vi "Get Plugin Paths.vi"(8 "error in":errorcluster, 11 "measurement customizations in":refnum<class "Measurement Plugin.lvclass">) -> (0 "error out":errorcluster, 2 "plugin paths":T1, 3 "measurement customizations out":refnum<class "Measurement Plugin.lvclass">)   [LabVIEW 2021, in "NIDAQmxMeasurement.lvlib" / "Measurement Plugin.lvclass"]
uses:
  Measurement Plugin.lvclass
  <vilib>/Plug-In SDKs/Measurements/Measurement Plugin Service/Plugin Paths.ctl
  Get Service Descriptor.vi
  Measurement Logic.vi
  Get UI Details.vi
  Measurement Configuration.ctl
  Measurement Results.ctl
  Get Type Specializations.vi
  Measurement Plugin.lvclass/Measurement Plugin.ctl
  NIDAQmxMeasurement.lvlib
  <vilib>/Plug-In SDKs/Measurements/Measurement Plugin Service/Measurement Plugin Service.lvclass
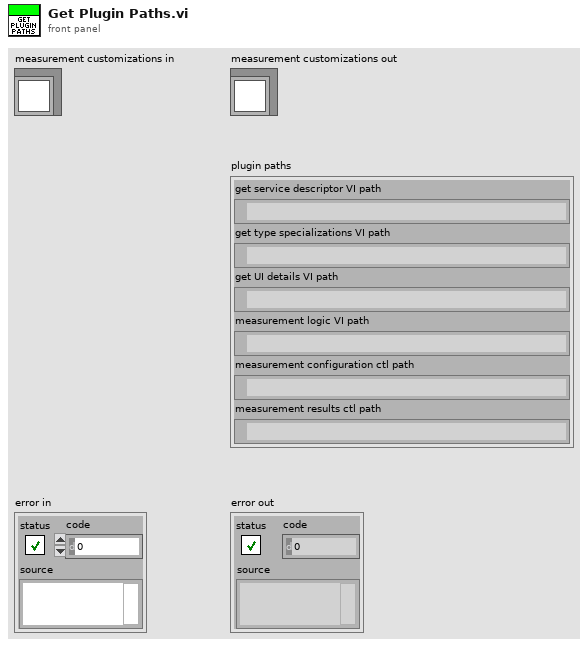
[diagram p1: front panel]
types:
  T1 = typedef "NI Measurement Plug-In SDK.lvlib/Measurement Plugin Service.lvclass/Plugin Paths.ctl" = cluster{"get service descriptor VI path":path, "get type specializations VI path":path, "get UI details VI path":path, "measurement logic VI path":path, "measurement configuration ctl path":path, "measurement results ctl path":path}
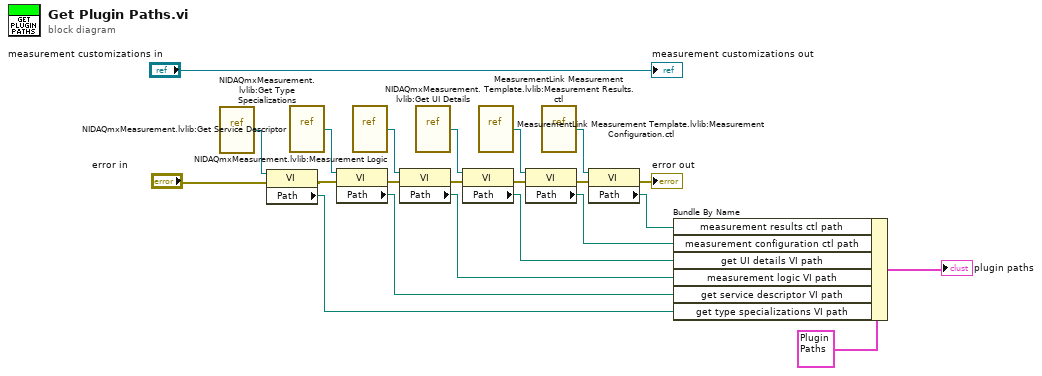
[diagram p0: block diagram]
diagram:
  n1 = vi-ref "NIDAQmxMeasurement.lvlib:Get Type Specializations.vi"() -> (w11:refnum<vi>)
  n2 = property class="VI"(reference=w11, error in="error in") -> (error out=w10:errorcluster, "Path"=w7:path)  [unwired: 1 out]
  n3 = vi-ref "NIDAQmxMeasurement.lvlib:Get Service Descriptor.vi"() -> (w12:refnum<vi>)
  n4 = property class="VI"(reference=w12, error in=w10) -> (error out=w17:errorcluster, "Path"=w5:path)  [unwired: 1 out]
  n5 = vi-ref "NIDAQmxMeasurement.lvlib:Measurement Logic.vi"() -> (w21:refnum<vi>)
  n6 = property class="VI"(reference=w21, error in=w17) -> (error out=w16:errorcluster, "Path"=w4:path)  [unwired: 1 out]
  n7 = vi-ref "NIDAQmxMeasurement.lvlib:Get UI Details.vi"() -> (w20:refnum<vi>)
  n8 = property class="VI"(reference=w20, error in=w16) -> (error out=w15:errorcluster, "Path"=w3:path)  [unwired: 1 out]
  n9 = vi-ref "MeasurementLink Measurement Template.lvlib:Measurement Configuration.ctl"() -> (w19:refnum<vi>)
  n10 = property class="VI"(reference=w19, error in=w15) -> (error out=w14:errorcluster, "Path"=w2:path)  [unwired: 1 out]
  n11 = vi-ref "MeasurementLink Measurement Template.lvlib:Measurement Results.ctl"() -> (w18:refnum<vi>)
  n12 = property class="VI"(reference=w18, error in=w14) -> (error out=→"error out":errorcluster, "Path"=w1:path)  [unwired: 1 out]
  n13 = Bundle By Name(cluster=T1 {"get service descriptor VI path"=path "", "get type specializations VI path"=path "", "get UI details VI path"=path "", "measurement logic VI path"=path "", "measurement configuration ctl path"=path "", "measurement results ctl path"=path ""} ("Plugin Paths"), "measurement results ctl path"=w1, "measurement configuration ctl path"=w2, "get UI details VI path"=w3, "measurement logic VI path"=w4, "get service descriptor VI path"=w5, "get type specializations VI path"=w7) -> (→"plugin paths":T1)
  "measurement customizations out" <- "measurement customizations in"
